vi "Launch Asynchronous VI.vi"(8 "error in (no error)":errorcluster, 10 "VI path":path) -> (0 "error out":errorcluster)   [LabVIEW 2011]
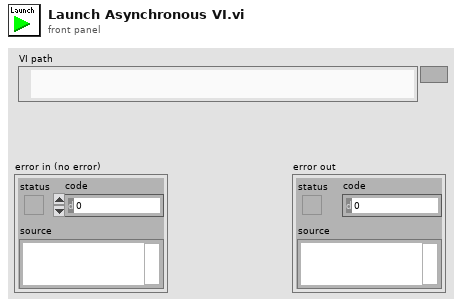
[diagram p1: front panel]
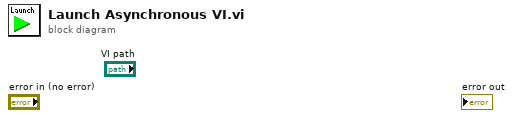
[diagram p0: block diagram]
diagram:
